vi "Laboratory_practice11.vi"() -> ()   [LabVIEW 2023]
panel:
  in  "rate":dbl=5000.0
  in  "number of samples":i32=100
  out "data":dynamicdata(graph)
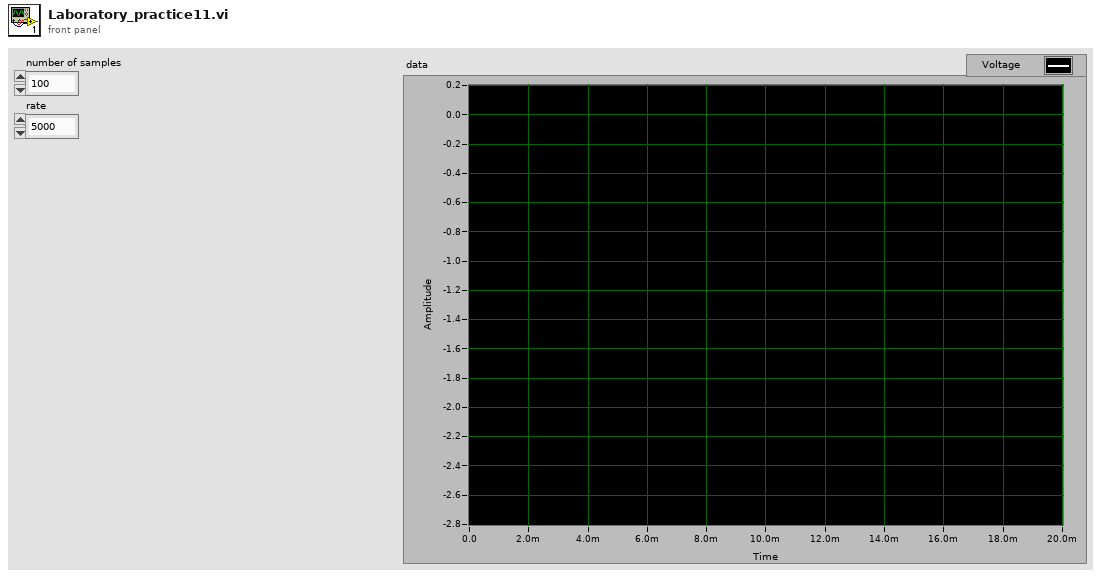
[diagram p1: front panel]
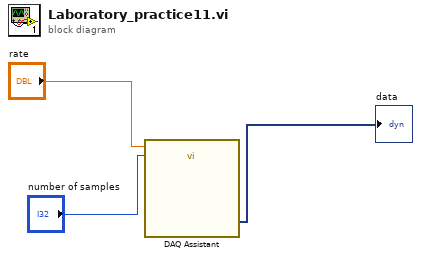
[diagram p0: block diagram]
diagram:
  n1 = call "DAQ Assistant"("rate"="rate", "number of samples"="number of samples") -> ("data"=→"data":dynamicdata)  [unwired: 15 in, 2 out]
